vi "MD5 Message Digest (Binary String)__ogtk.vi"(1 "Message":string) -> (0 "MD5 Message Digest":string)   [LabVIEW 2012]
doc: "Implements the MD5 algorithm to produce a 128-Bit Hash condensed representation of a message or a data file.\n\nPolymorphic VI can output MD5 Hash as Binary String or Hexadeximal String."
panel:
  # "Please visit http://www.OpenG.org to learn about the\nOpen Source LabVIEW software movement.\n\nNOTICE -- YOU MUST LEAVE THIS NOTICE IN PLACE.  PER THE TERMS OF THE LICENSE BELOW, YOU MAY SUBLICENSE THIS SOFTWARE \nIN ANY WAY THAT DOES NOT CONFLICT WITH THIS LICENSE.\n\n### BSD License (http://www.opensource.org/licenses/bsd-license.php) Begin ###\n \nCopyright (c) 2004, Enrique Vargas <vargas@visecurity.com>\nCopyright (c) 2011, Jonathon Green <jg@jgcode.net>\n\nAll rights reserved.\n\nRedistribution and use in source and binary forms, with or without modification, are permitted provided that the following conditions are met:\n\n    * Redistributions of source code must retain the above copyright notice, this list of conditions and the following disclaimer.\n    * Redistributions in binary form must reproduce the above copyright notice, this list of conditions and the following disclaimer in the \n       documentation and/or other materials provided with the distribution.\n    * Neither the name of SciWare, James Kring, Inc., nor the names of its contributors may be used to endorse or promote products derived \n       from this software without specific prior written permission.\n\nTHIS SOFTWARE IS PROVIDED BY THE COPYRIGHT HOLDERS AND CONTRIBUTORS \"AS IS\" AND ANY EXPRESS OR IMPLIED WARRANTIES, \nINCLUDING, BUT NOT LIMITED TO, THE IMPLIED WARRANTIES OF MERCHANTABILITY AND FITNESS FOR A PARTICULAR PURPOSE ARE \nDISCLAIMED. IN NO EVENT SHALL THE COPYRIGHT OWNER OR CONTRIBUTORS BE LIABLE FOR ANY DIRECT, INDIRECT, INCIDENTAL,\n SPECIAL, EXEMPLARY, OR CONSEQUENTIAL DAMAGES (INCLUDING, BUT NOT LIMITED TO, PROCUREMENT OF SUBSTITUTE GOODS OR \nSERVICES; LOSS OF USE, DATA, OR PROFITS; OR BUSINESS INTERRUPTION) HOWEVER CAUSED AND ON ANY THEORY OF LIABILITY, \nWHETHER IN CONTRACT, STRICT LIABILITY, OR TORT (INCLUDING NEGLIGENCE OR OTHERWISE) ARISING IN ANY WAY OUT OF THE USE \nOF THIS SOFTWARE, EVEN IF ADVISED OF THE POSSIBILITY OF SUCH DAMAGE.\n\n### BSD License End ###"
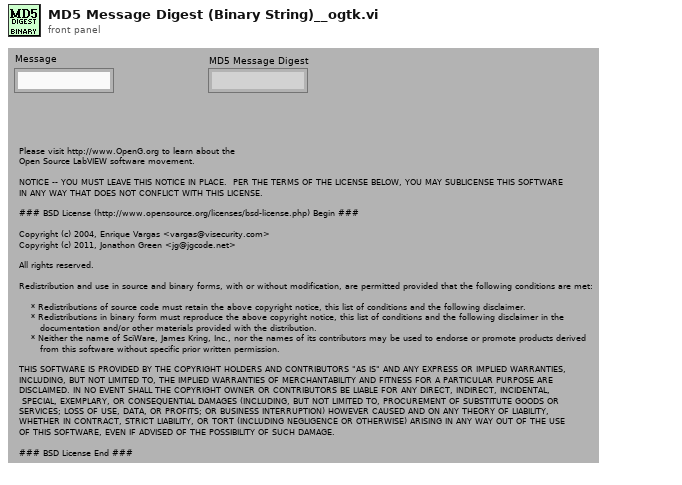
[diagram p1: front panel]
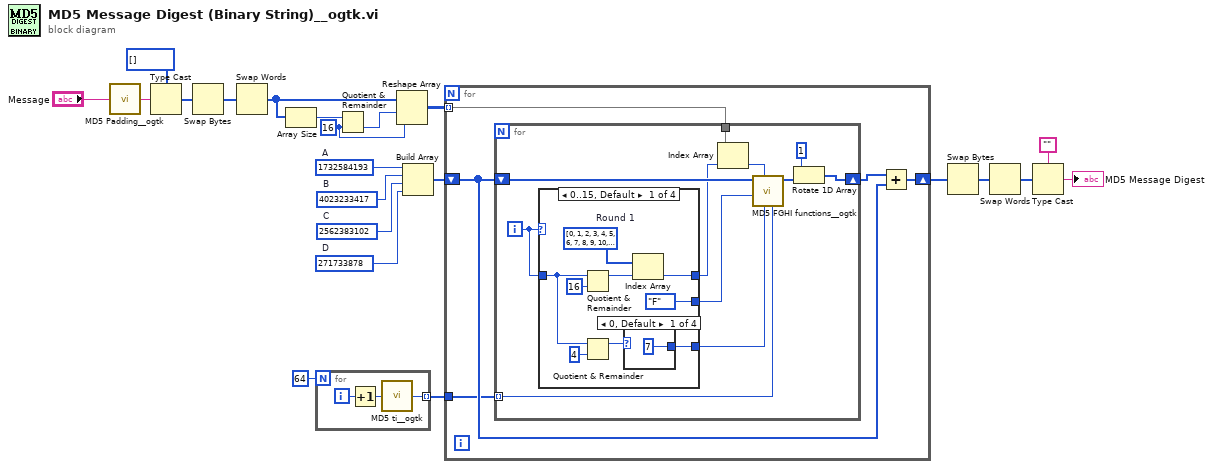
[diagram p0: block diagram]
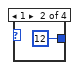
[diagram p2: hidden frame]
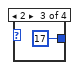
[diagram p3: hidden frame]
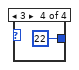
[diagram p4: hidden frame]
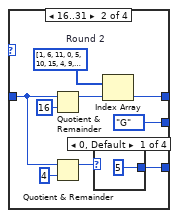
[diagram p5: hidden frame]
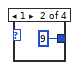
[diagram p6: hidden frame]
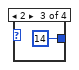
[diagram p7: hidden frame]
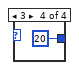
[diagram p8: hidden frame]
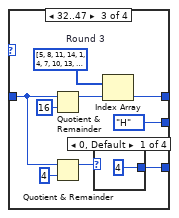
[diagram p9: hidden frame]
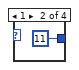
[diagram p10: hidden frame]
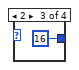
[diagram p11: hidden frame]
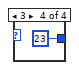
[diagram p12: hidden frame]
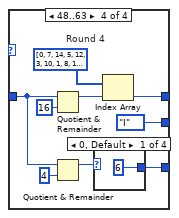
[diagram p13: hidden frame]
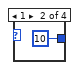
[diagram p14: hidden frame]
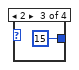
[diagram p15: hidden frame]
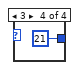
[diagram p16: hidden frame]
diagram:
  w16 = u32 1732584193  # A
  w15 = u32 4023233417  # B
  w14 = u32 2562383102  # C
  w13 = u32 271733878  # D
  w10 = 16 ("y")
  n1 = call <userlib>:"MD5 Padding__ogtk.vi"("String"="Message") -> ("MD5 Padded String"=w22:string)
  n2 = Type Cast(type=u32[] [] ("Array Constant"), x=w22) -> (*(type *) &x=w8:u32[])
  n3 = Swap Bytes(anything=w8) -> (byte swapped=w6:u32[])
  n4 = Swap Words(1:w6) -> (0:w5:u32[])
  n5 = Array Size(array=w5) -> (size(s)=w20:i32)
  n6 = for {
    N: 64 -> [_]
    tunnel: [w23] -> w1 mode=indexing
    i -> [w24]
    n7 = Increment(x=w24) -> (x+1=w25:i32)
    n8 = call <userlib>:"MD5 ti__ogtk.vi"("i"=w25) -> ("ti"=w23:u32)
  }
  n9 = Quotient & Remainder(x=w20, y=w10) -> (floor(x/y)=w11:i32)  [unwired: 1 out]
  n10 = Reshape Array(w5, w11, w10) -> (w9:u32[][])
  n11 = Build Array(w16, w15, w14, w13) -> (w12:u32[])
  n12 = for {
    shift-right: [w29] -> w7
    shift-left: w12 -> [w30]
    tunnel: w9 -> [w27] mode=indexing
    tunnel: w1 -> [w26]
    n13 = for {
      tunnel: w27 -> [w35]
      shift-right: [w40] -> w28
      shift-left: w30 -> [w38]
      tunnel: w26 -> [w31] mode=indexing
      i -> [w39]
      n14 = case shown="0..15, Default" w39 {
        tunnel: w39 -> [w47 w61 w74 w87]
        tunnel: [enum16{"F", "G", "H", "I"}."F" ("Operator function") enum16{"F", "G", "H", "I"}."G" ("Operator function") enum16{"F", "G", "H", "I"}."H" ("Operator function") enum16{"F", "G", "H", "I"}."I" ("Operator function")] -> w33
        tunnel: [w43 w56 w69 w82] -> w32
        tunnel: [w42 w55 w68 w81] -> w36
        frame 0..15, Default {
          w46 = i32[] [0, 1, 2, 3, 4, 5, 6, 7, 8, 9, 10, 11, 12, 13, 14, 15]  # Round 1
          n15 = Quotient & Remainder(x=w47, y=16) -> (x-y*floor(x/y)=w45:i32)  [unwired: 1 out]
          n16 = Quotient & Remainder(x=w47, y=4) -> (x-y*floor(x/y)=w49:i32)  [unwired: 1 out]
          n17 = case shown="0, Default" w49 {
            tunnel: [7 ("s") 12 ("s") 17 ("s") 22 ("s")] -> w43
            frame 0, Default {
            }
            frame 1 {
            }
            frame 2 {
            }
            frame 3 {
            }
          }
          n18 = Index Array(array=w46, index=w45) -> (element=w42:i32)
        }
        frame 16..31 {
          w59 = i32[] [1, 6, 11, 0, 5, 10, 15, 4, 9, 14, 3, 8, 13, 2, 7, 12]  # Round 2
          n19 = Quotient & Remainder(x=w61, y=16) -> (x-y*floor(x/y)=w60:i32)  [unwired: 1 out]
          n20 = Quotient & Remainder(x=w61, y=4) -> (x-y*floor(x/y)=w58:i32)  [unwired: 1 out]
          n21 = case shown="0, Default" w58 {
            tunnel: [5 ("s") 9 ("s") 14 ("s") 20 ("s")] -> w56
            frame 0, Default {
            }
            frame 1 {
            }
            frame 2 {
            }
            frame 3 {
            }
          }
          n22 = Index Array(array=w59, index=w60) -> (element=w55:i32)
        }
        frame 32..47 {
          w72 = i32[] [5, 8, 11, 14, 1, 4, 7, 10, 13, 0, 3, 6, 9, 12, 15, 2]  # Round 3
          n23 = Quotient & Remainder(x=w74, y=16) -> (x-y*floor(x/y)=w73:i32)  [unwired: 1 out]
          n24 = Quotient & Remainder(x=w74, y=4) -> (x-y*floor(x/y)=w71:i32)  [unwired: 1 out]
          n25 = case shown="0, Default" w71 {
            tunnel: [4 ("s") 11 ("s") 16 ("s") 23 ("s")] -> w69
            frame 0, Default {
            }
            frame 1 {
            }
            frame 2 {
            }
            frame 3 {
            }
          }
          n26 = Index Array(array=w72, index=w73) -> (element=w68:i32)
        }
        frame 48..63 {
          w85 = i32[] [0, 7, 14, 5, 12, 3, 10, 1, 8, 15, 6, 13, 4, 11, 2, 9]  # Round 4
          n27 = Quotient & Remainder(x=w87, y=16) -> (x-y*floor(x/y)=w86:i32)  [unwired: 1 out]
          n28 = Quotient & Remainder(x=w87, y=4) -> (x-y*floor(x/y)=w84:i32)  [unwired: 1 out]
          n29 = case shown="0, Default" w84 {
            tunnel: [6 ("s") 10 ("s") 15 ("s") 21 ("s")] -> w82
            frame 0, Default {
            }
            frame 1 {
            }
            frame 2 {
            }
            frame 3 {
            }
          }
          n30 = Index Array(array=w85, index=w86) -> (element=w81:i32)
        }
      }
      n31 = Index Array(array=w35, index=w36) -> (element=w34:u32)
      n32 = call <userlib>:"MD5 FGHI functions__ogtk.vi"("ti"=w31, "s"=w32, "Mj"=w34, "Operator function"=w33, "Chaining Variables"=w38) -> ("Resulting Chaining Variables"=w37:u32[])  [unwired: 6 in]
      n33 = Rotate 1D Array(1:w37, 2:1 ("n")) -> (0:w40:u32[])
    }
    n34 = Add(x=w28, y=w30) -> (x+y=w29:u32[])
  }
  n35 = Swap Bytes(anything=w7) -> (byte swapped=w4:u32[])
  n36 = Swap Words(1:w4) -> (0:w3:u32[])
  n37 = Type Cast(type="", x=w3) -> (*(type *) &x=→"MD5 Message Digest":string)
